vi "Filter-Apply.vi"(0 "Filter":T1 {"IIR Filter Cluster"."Forward Coefficients" format="%.4f"; "IIR Filter Cluster"."Reverse Coefficients" format="%.4f"}, 7 "X":dbl[](array[numeric]), 11 "error in (no error)":errorcluster) -> (4 "Filter out":T1 {"IIR Filter Cluster"."Forward Coefficients" format="%.4f"; "IIR Filter Cluster"."Reverse Coefficients" format="%.4f"}, 8 "Filtered X":dbl[](array[numeric]), 15 "error out":errorcluster)   [LabVIEW 2020]
uses:
  Controls/Filter XCtl/Filter Data.ctl
  <vilib>/Analysis/3filter.llb/IIR Cascade Filter with I.C. (DBL).vi
  <vilib>/Analysis/NI_AALBase.lvlib
  <vilib>/Analysis/NI_AALPro.lvlib
  Controls/Filter XCtl/Filter XCtl.xctl
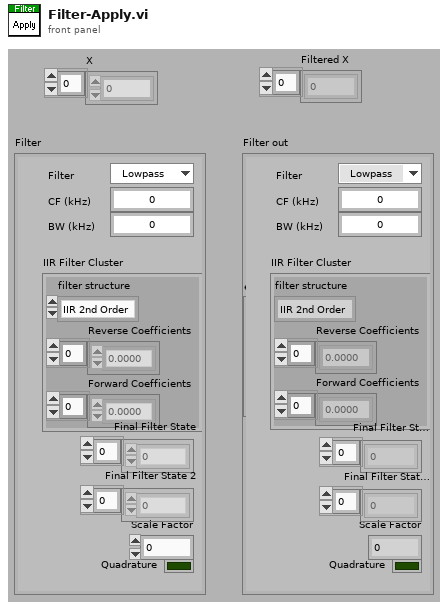
[diagram p1: front panel]
types:
  T1 = typedef "Filter XCtl.xctl/Filter Data.ctl" = cluster{"CF (kHz)":dbl, "BW (kHz)":dbl, "IIR Filter Cluster":cluster{"filter structure":enum32{"IIR 2nd Order", "IIR 4th Order"}, "Reverse Coefficients":dbl[], "Forward Coefficients":dbl[]}, "Final Filter State":dbl[], "Scale Factor":dbl, "Final Filter State 2":dbl[], "Quadrature":bool, "Type":enum16{"Lowpass", "Highpass", "Bandpass", "Bandstop", "OFF"}}
  T2 = cluster{"filter structure":enum32{"IIR 2nd Order", "IIR 4th Order"}, "Reverse Coefficients":dbl[], "Forward Coefficients":dbl[]}
  T3 = enum16{"Lowpass", "Highpass", "Bandpass", "Bandstop", "OFF"}
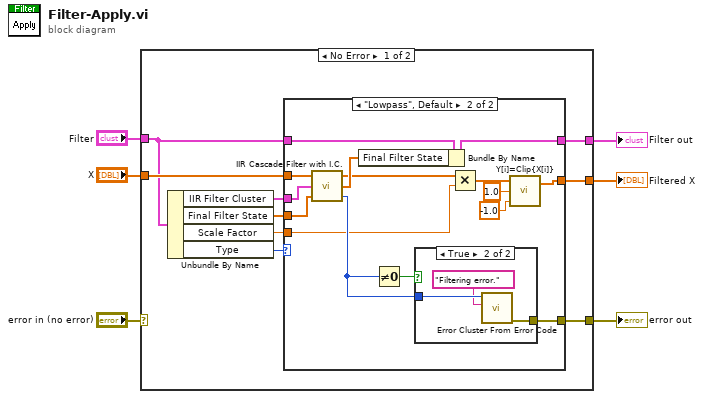
[diagram p0: block diagram]
diagram:
  n1 = case shown="No Error" "error in (no error)" {
    selector: "error in (no error)" -> [_ w38]
    tunnel: "X" -> [w15 w37]
    tunnel: "Filter" -> [w12 w36]
    tunnel: [w11 w38] -> w4
    tunnel: [w9 w37] -> w2
    tunnel: [w8 w36] -> w1
    frame No Error {
      n2 = Unbundle By Name(w12) -> ("IIR Filter Cluster"=w14:T2, "Final Filter State"=w13:dbl[], "Scale Factor"=w7:dbl, "Type"=w10:T3)
      n3 = case shown="\"Lowpass\", Default" w10 {
        tunnel: w15 -> [w17 w32]
        tunnel: w14 -> [_ w31]
        tunnel: w13 -> [_ w22]
        tunnel: w12 -> [w16 w30]
        tunnel: [_ w28] -> w11
        tunnel: [w17 w20] -> w9
        tunnel: [w16 w26] -> w8
        tunnel: w7 -> [_ w23]
        frame "OFF" {
        }
        frame "Lowpass", Default {
          n4 = call-poly <vilib>:"IIR Cascade Filter with I.C..vi"("Initial Filter State"=w22, "IIR Filter Cluster"=w31, "X"=w32) -> ("error"=w27:i32, "Final Filter State"=w25:dbl[], "Filtered X"=w24:dbl[])
          n5 = Bundle By Name(cluster=w30, "Final Filter State"=w25) -> (w26:T1)
          n6 = Not Equal To 0?(x=w27) -> (x != 0?=w29:bool)
          n7 = case shown="True" w29 {
            tunnel: [_ w34] -> w28
            tunnel: w27 -> [_ w35]
            frame False {
            }
            frame True {
              n8 = call <vilib>:"Error Cluster From Error Code.vi"("error message (\"\")"="Filtering error." ("error message (\"\")"), "error code (0)"=w35) -> ("error out"=w34:errorcluster)  [unwired: 7 in]
            }
          }
          n9 = Multiply(x=w24, y=w23) -> (x*y=w21:dbl[])
          n10 = call <vilib>:"Y[i]=Clip{X[i]}.vi"("lower limit"=-1.0, "upper limit"=1.0, "Input Array"=w21) -> ("Clipped Array"=w20:dbl[])  [unwired: 1 out]
        }
      }
    }
    frame Error {
    }
  }
  "error out" <- w4
  "Filtered X" <- w2
  "Filter out" <- w1
